vi "Day11-02.vi"() -> ()   [LabVIEW 2021]
uses:
  <vilib>/DAQmx/read.llb/DAQmx Read (Analog 2D DBL NChan NSamp).vi
  <vilib>/DAQmx/create/channels.llb/DAQmx Create Channel (AI-Voltage-Basic).vi
  <vilib>/DAQmx/configure/timing.llb/DAQmx Timing (Sample Clock).vi
  <vilib>/DAQmx/miscellaneous.llb/DAQmx Fill In Error Info.vi
panel:
  out "전치된 배열 2":dbl[][](graph)
  out "전치된 배열":dbl[][](array[numeric])
  out "최대값":dbl
  in  "정지":bool
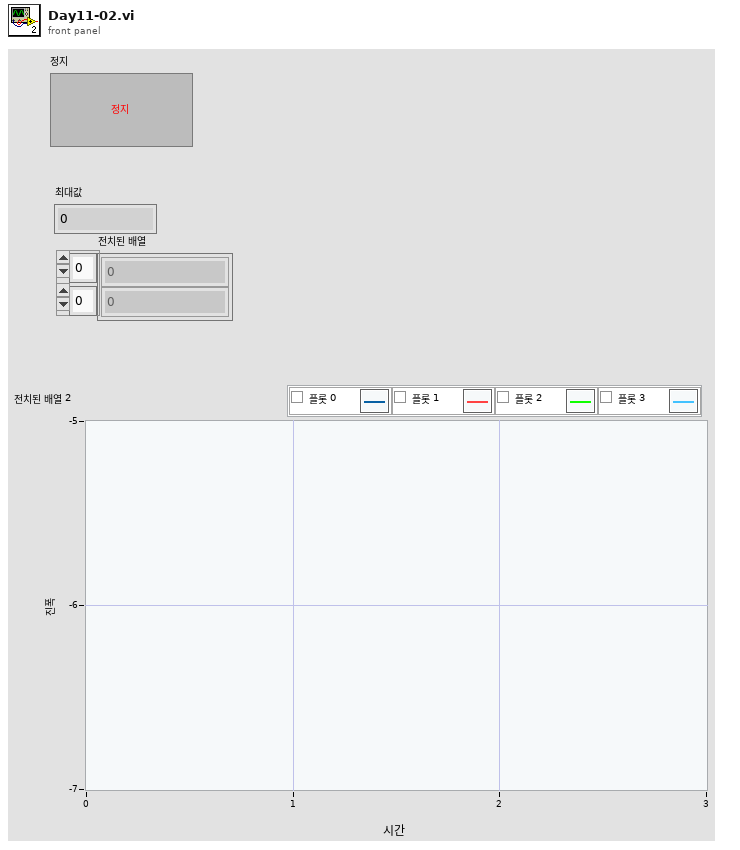
[diagram p1: front panel]
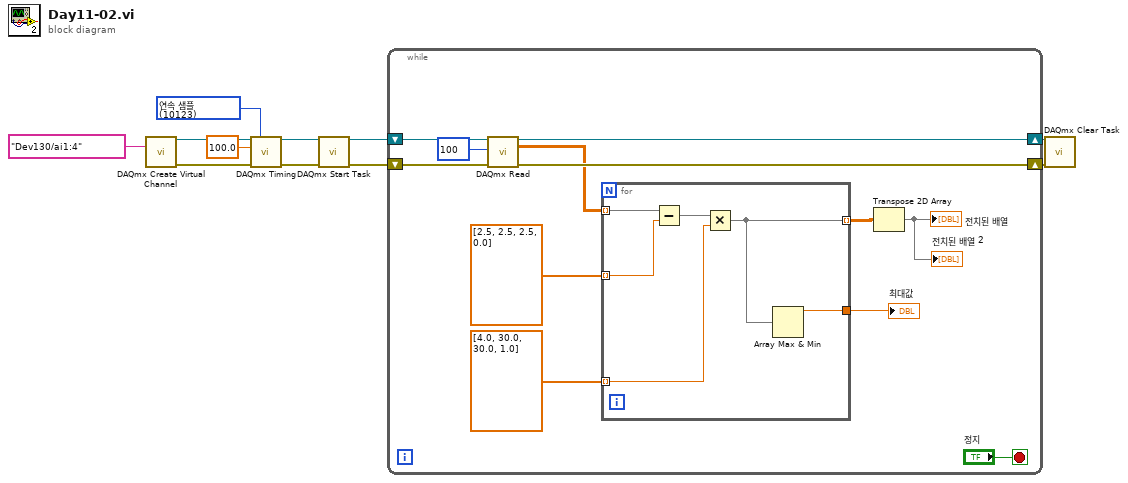
[diagram p0: block diagram]
diagram:
  w2 = 10123 items=["유한 샘플"=10178, "연속 샘플"=10123, "하드웨어 타이밍에 의한 단일 포인트"=12522] ("sample mode")
  n1 = call-poly <vilib>:"DAQmx Create Virtual Channel.vi"("physical channels"=tag "Dev130/ai1:4") -> ("task out"=w11:refnum<k21>, "error out"=w10:errorcluster)  [unwired: 13 in]
  n2 = call-poly <vilib>:"DAQmx Timing.vi"("task/channels in"=w11, "sample mode"=w2, "rate"=100.0, "error in"=w10) -> ("task out"=w9:refnum<k21>, "error out"=w8:errorcluster)  [unwired: 10 in]
  n3 = call <vilib>:"DAQmx Start Task.vi"("task/channels in"=w9, "error in"=w8) -> ("task out"=w7:refnum<k21>, "error out"=w6:errorcluster)  [unwired: 12 in]
  n4 = while {
    shift-right: [w21] -> w5
    shift-left: w7 -> [w23]
    shift-right: [w20] -> w4
    shift-left: w6 -> [w22]
    stop <- "정지" stop-if-true
    n5 = call-poly <vilib>:"DAQmx Read.vi"("task/channels in"=w23, "number of samples per channel"=100, "error in"=w22) -> ("task out"=w21:refnum<k21>, "data"=w17:dbl[][], "error out"=w20:errorcluster)  [unwired: 10 in]
    n6 = for {
      tunnel: w17 -> [w29] mode=indexing
      tunnel: dbl[] [2.5, 2.5, 2.5, 0.0] ("y") -> [w28] mode=indexing
      tunnel: dbl[] [4.0, 30.0, 30.0, 1.0] ("y") -> [w27] mode=indexing
      tunnel: [w25] -> w13 mode=indexing
      tunnel: [w24] -> w14
      n7 = Subtract(x=w29, y=w28) -> (x-y=w26:dbl[])
      n8 = Multiply(x=w26, y=w27) -> (x*y=w25:dbl[])
      n9 = Array Max & Min(array=w25) -> (max value=w24:dbl)  [unwired: 3 out]
    }
    "최대값" <- w14
    n10 = Transpose 2D Array(2D array=w13) -> (transposed array=→"전치된 배열" →"전치된 배열 2":dbl[][])
  }
  n11 = call <vilib>:"DAQmx Clear Task.vi"("task in"=w5, "error in"=w4) -> ()  [unwired: 13 in, 1 out]
